vi "Inclusion_main.vi"() -> ()   [LabVIEW 2018]
uses:
  <userlib>/_OpenG.lib/numeric/numeric.llb/Random Number Within Range - DBL__ogtk.vi
  <vilib>/Analysis/NI_AALBase.lvlib
panel:
  out "Histogram Graph":T1(graph)
  out "Avg. us per sample":dbl
  in  "N samples":i32=1000
  in  "Test":bool
  in  "Type":bool
  out "Reset c3":bool
  out "Reset c2":bool
  out "Reset c1":bool
  out "Out 3":dbl
  out "Out 2":dbl
  in  "Send 3":dbl
  in  "Send 2":dbl
  out "Out 1":dbl
  in  "Send 1":dbl
  in  "Stop Button":bool
  in  "Reset all":bool
  in  "Send":bool
  in  "Reset 3":bool
  in  "Reset 2":bool
  in  "Reset 1":bool
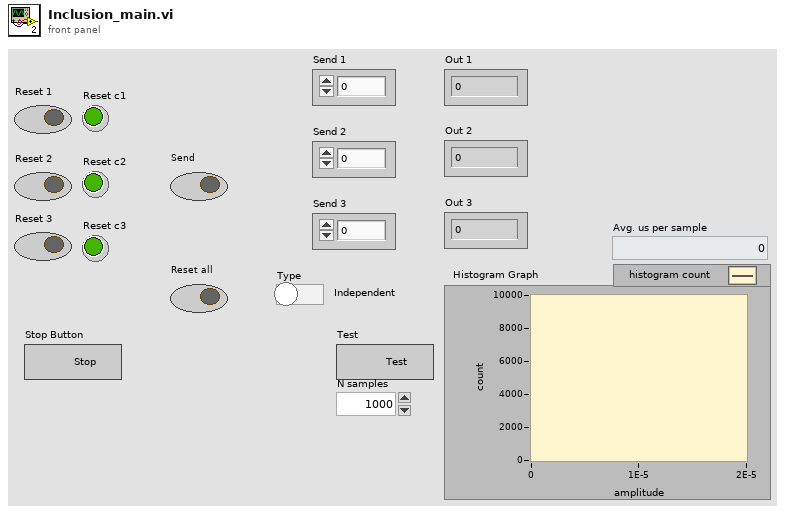
[diagram p1: front panel]
types:
  T1 = cluster{"X Values":dbl[], "Histogram: h(x)":i32[]}
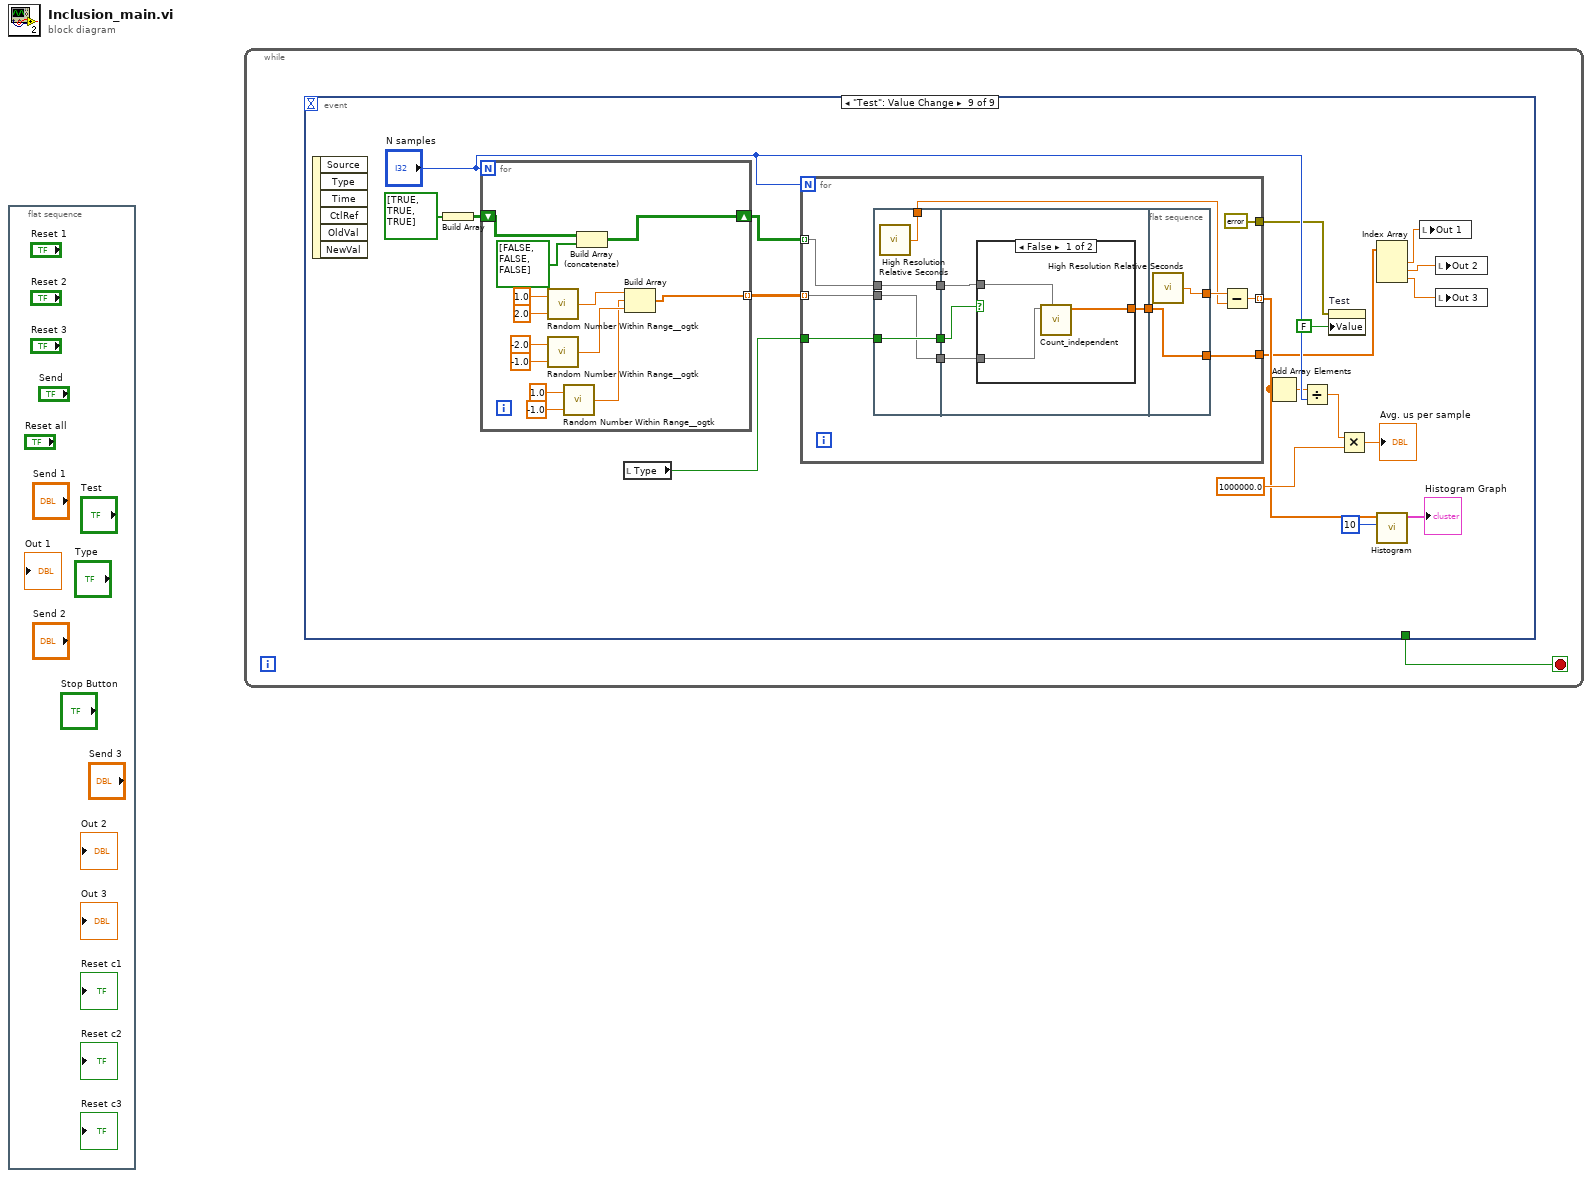
[diagram p0: block diagram]
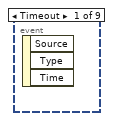
[diagram p2: hidden frame]
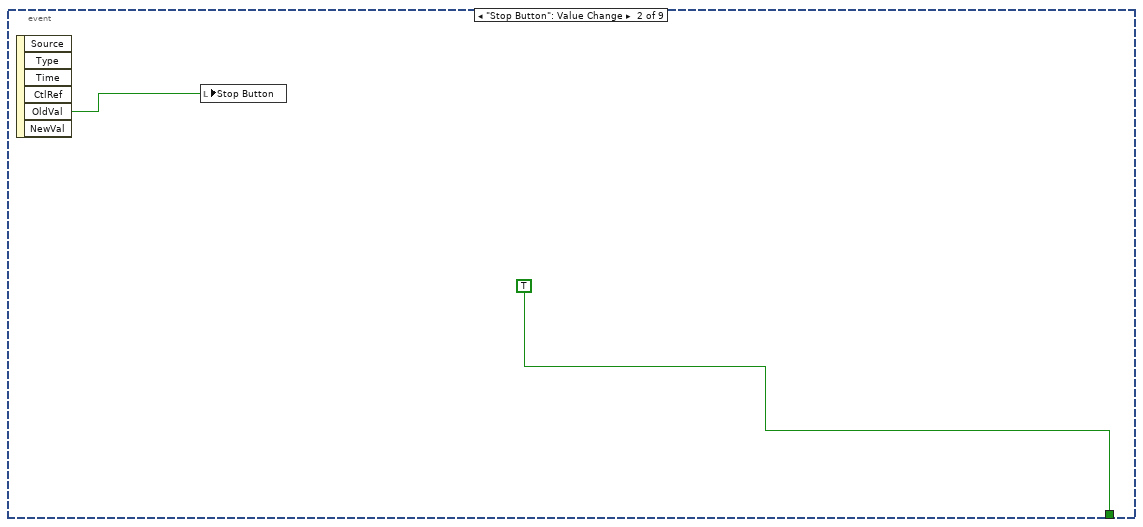
[diagram p3: hidden frame]
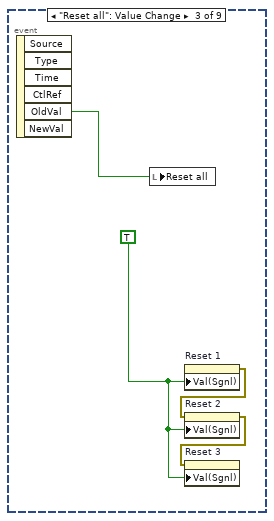
[diagram p4: hidden frame]
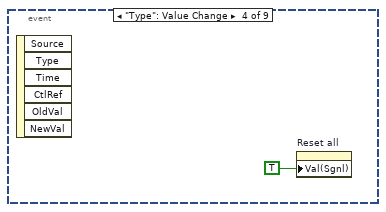
[diagram p5: hidden frame]
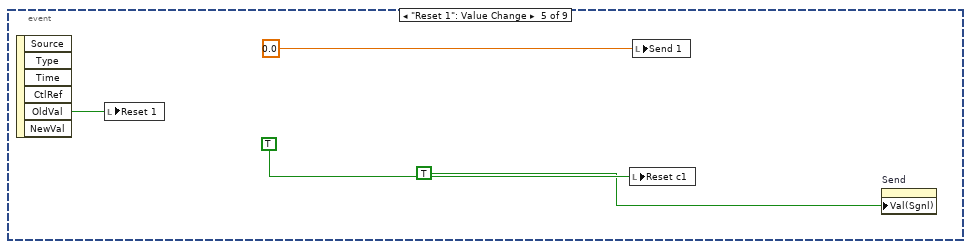
[diagram p6: hidden frame]
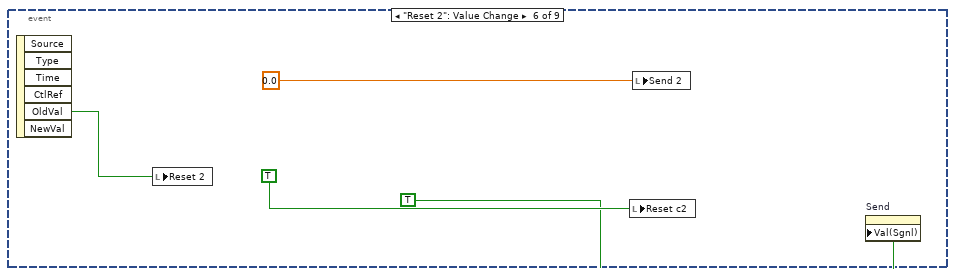
[diagram p7: hidden frame]
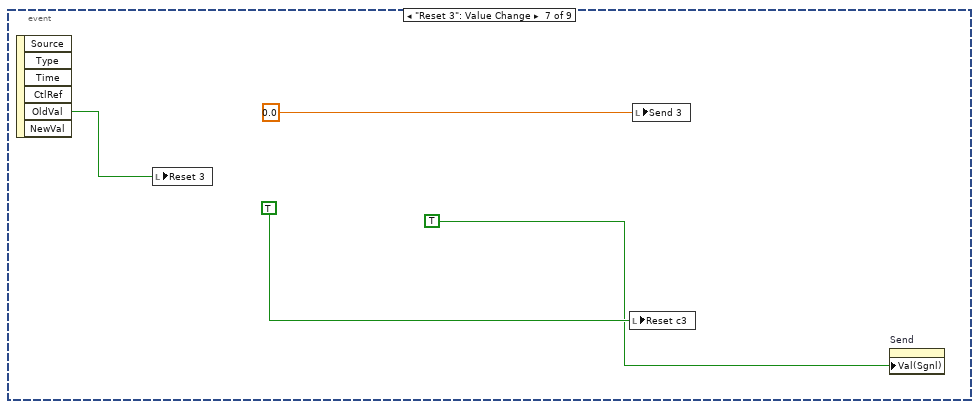
[diagram p8: hidden frame]
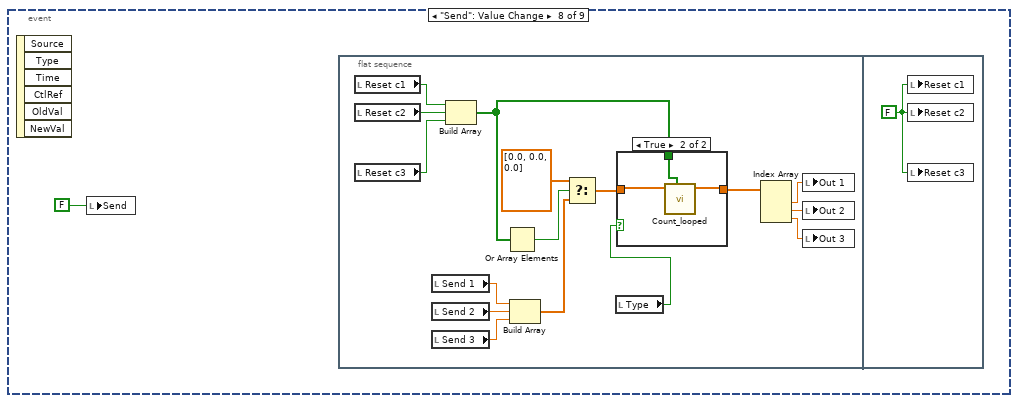
[diagram p9: hidden frame]
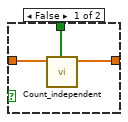
[diagram p10: hidden frame]
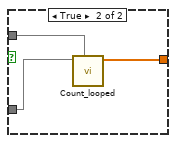
[diagram p11: hidden frame]
diagram:
  n1 = flat-sequence {
    frame #0 {
    }
  }
  n2 = while {
    stop <- w1 stop-if-true
    n3 = event shown="[8] \"Test\": Value Change" {
      selector: _ -> [_ _ _ _ _ _ _ _ _]
      dyn-events: _ -> [_ _ _ _ _ _ _ _ _]
      timeout: _ -> [_ _ _ _ _ _ _ _ _]
      tunnel: [_ TRUE _ _ _ _ _ _ _] -> w1
      event Timeout {
        n4 = event-data() -> ()  [unwired: 1 in, 3 out]
      }
      event "Stop Button": Value Change {
        n5 = event-data() -> ("OldVal"=w2:bool)  [unwired: 1 in, 5 out]
        n6 = local write "Stop Button"(w2) -> ()
      }
      event "Reset all": Value Change {
        w6 = TRUE ("Value (Signaling)")
        n7 = event-data() -> ("OldVal"=w7:bool)  [unwired: 1 in, 5 out]
        n8 = local write "Reset all"(w7) -> ()
        n9 = property on="Reset 1" class="Bool (strict)"("Val(Sgnl)"=w6) -> (error out=w5:errorcluster)  [unwired: 2 in, 1 out]
        n10 = property on="Reset 2" class="Bool (strict)"(error in=w5, "Val(Sgnl)"=w6) -> (error out=w4:errorcluster)  [unwired: 1 in, 1 out]
        n11 = property on="Reset 3" class="Bool (strict)"(error in=w4, "Val(Sgnl)"=w6) -> ()  [unwired: 1 in, 2 out]
      }
      event "Type": Value Change {
        n12 = event-data() -> ()  [unwired: 1 in, 6 out]
        n13 = property on="Reset all" class="Bool (strict)"("Val(Sgnl)"=TRUE ("Value (Signaling)")) -> ()  [unwired: 2 in, 2 out]
      }
      event "Reset 1": Value Change {
        n14 = event-data() -> ("OldVal"=w11:bool)  [unwired: 1 in, 5 out]
        n15 = local write "Reset 1"(w11) -> ()
        n16 = local write "Reset c1"(TRUE ("Reset c1")) -> ()
        n17 = local write "Send 1"(0.0 ("Send 1")) -> ()
        n18 = property on="Send" class="Bool (strict)"("Val(Sgnl)"=TRUE ("Value (Signaling)")) -> ()  [unwired: 2 in, 2 out]
      }
      event "Reset 2": Value Change {
        n19 = event-data() -> ("OldVal"=w15:bool)  [unwired: 1 in, 5 out]
        n20 = local write "Reset 2"(w15) -> ()
        n21 = local write "Reset c2"(TRUE ("Reset c2")) -> ()
        n22 = local write "Send 2"(0.0 ("Send 2")) -> ()
        n23 = property on="Send" class="Bool (strict)"("Val(Sgnl)"=TRUE ("Value (Signaling)")) -> ()  [unwired: 2 in, 2 out]
      }
      event "Reset 3": Value Change {
        n24 = event-data() -> ("OldVal"=w19:bool)  [unwired: 1 in, 5 out]
        n25 = local write "Reset 3"(w19) -> ()
        n26 = local write "Reset c3"(TRUE ("Reset c3")) -> ()
        n27 = local write "Send 3"(0.0 ("Send 3")) -> ()
        n28 = property on="Send" class="Bool (strict)"("Val(Sgnl)"=TRUE ("Value (Signaling)")) -> ()  [unwired: 2 in, 2 out]
      }
      event "Send": Value Change {
        n29 = event-data() -> ()  [unwired: 1 in, 6 out]
        n30 = local write "Send"(FALSE ("Send")) -> ()
        n31 = flat-sequence {
          frame #0 {
            n32 = local read "Reset c1"() -> (w30:bool)
            n33 = local read "Reset c2"() -> (w29:bool)
            n34 = local read "Reset c3"() -> (w28:bool)
            n35 = local read "Send 1"() -> (w37:dbl)
            n36 = local read "Send 2"() -> (w36:dbl)
            n37 = local read "Send 3"() -> (w35:dbl)
            n38 = Build Array(w30, w29, w28) -> (w27:bool[])
            n39 = Or Array Elements(Boolean array=w27) -> (logical OR=w24:bool)
            n40 = Build Array(w37, w36, w35) -> (w25:dbl[])
            n41 = Select(t=dbl[] [0.0, 0.0, 0.0], s=w24, f=w25) -> (s? t:f=w26:dbl[])
            n42 = local read "Type"() -> (w22:bool)
            n43 = case shown="True" w22 {
              tunnel: [w40 w42] -> w34
              tunnel: w27 -> [w39 w41]
              tunnel: w26 -> [w38 w43]
              frame False {
                n44 = call "Count_independent.vi"("Reset?"=w39, "Input array"=w38) -> ("Output array"=w40:dbl[])  [unwired: 9 in]
              }
              frame True {
                n45 = call "Count_looped.vi"("Reset?"=w41, "Input array"=w43) -> ("Output array"=w42:dbl[])  [unwired: 9 in]
              }
            }
            n46 = Index Array(array=w34) -> (element #1=w33:dbl, element #2=w32:dbl, element #3=w31:dbl)  [unwired: 3 in]
            n47 = local write "Out 1"(w33) -> ()
            n48 = local write "Out 2"(w32) -> ()
            n49 = local write "Out 3"(w31) -> ()
          }
          frame #1 {
            w44 = FALSE ("Reset c1")
            n50 = local write "Reset c1"(w44) -> ()
            n51 = local write "Reset c2"(w44) -> ()
            n52 = local write "Reset c3"(w44) -> ()
          }
        }
      }
      event "Test": Value Change {
        n53 = event-data() -> ()  [unwired: 1 in, 6 out]
        n54 = Build Array(bool[] [TRUE, TRUE, TRUE]) -> (w46:bool[][])
        n55 = for {
          N: "N samples" -> [_]
          tunnel: [w93] -> w51 mode=indexing
          shift-right: [w92] -> w45
          shift-left: w46 -> [w104]
          n56 = call-poly <userlib>:"Random Number Within Range__ogtk.vi"("High"=1.0, "Low"=2.0) -> ("Random Number"=w100:dbl)  [unwired: 3 in]
          n57 = call-poly <userlib>:"Random Number Within Range__ogtk.vi"("High"=-2.0, "Low"=-1.0) -> ("Random Number"=w97:dbl)  [unwired: 3 in]
          n58 = call-poly <userlib>:"Random Number Within Range__ogtk.vi"("High"=1.0, "Low"=-1.0) -> ("Random Number"=w94:dbl)  [unwired: 3 in]
          n59 = Build Array (concatenate)(w104, bool[] [FALSE, FALSE, FALSE]) -> (w92:bool[][])
          n60 = Build Array(w100, w94, w97) -> (w93:dbl[])
        }
        n61 = local read "Type"() -> (w54:bool)
        n62 = for {
          N: "N samples" -> [_]
          tunnel: [w73] -> w57 mode=indexing
          tunnel: w54 -> [w71]
          tunnel: [errorcluster {"status"=FALSE, "code"=0, "source"=""} ("error in (no error)")] -> w52
          tunnel: w51 -> [w66] mode=indexing
          tunnel: w45 -> [w68] mode=indexing
          tunnel: [w65] -> w50
          n63 = flat-sequence {
            tunnel: [w79] -> w74
            tunnel: [w78] -> w72
            tunnel: w71 -> [w78]
            tunnel: [w77] -> w69
            tunnel: w68 -> [w77]
            tunnel: [w76] -> w67
            tunnel: w66 -> [w76]
            tunnel: w72 -> [w83]
            tunnel: w69 -> [w82]
            tunnel: w67 -> [w81]
            tunnel: [w80] -> w64
            tunnel: [w91] -> w75
            tunnel: [w90] -> w65
            tunnel: w64 -> [w90]
            frame #0 {
              n64 = call <vilib>:"High Resolution Relative Seconds.vi"() -> ("relative seconds"=w79:dbl)
            }
            frame #1 {
              n65 = case shown="False" w83 {
                tunnel: w82 -> [w86 w88]
                tunnel: w81 -> [w85 w89]
                tunnel: [w84 w87] -> w80
                frame False {
                  n66 = call "Count_independent.vi"("Reset?"=w86, "Input array"=w85) -> ("Output array"=w84:dbl[])  [unwired: 9 in]
                }
                frame True {
                  n67 = call "Count_looped.vi"("Reset?"=w88, "Input array"=w89) -> ("Output array"=w87:dbl[])  [unwired: 9 in]
                }
              }
            }
            frame #2 {
              n68 = call <vilib>:"High Resolution Relative Seconds.vi"() -> ("relative seconds"=w91:dbl)
            }
          }
          n69 = Subtract(x=w75, y=w74) -> (x-y=w73:dbl)
        }
        n70 = Add Array Elements(numeric array=w57) -> (sum=w60:dbl)
        n71 = Divide(x=w60, y="N samples") -> (x/y=w61:dbl)
        n72 = property on="Test" class="Bool (strict)"(error in=w52, "Value"=FALSE ("Test")) -> ()  [unwired: 1 in, 2 out]
        n73 = Multiply(x=w61, y=1000000.0) -> (x*y=→"Avg. us per sample":dbl)
        n74 = Index Array(array=w50) -> (element #1=w49:dbl, element #2=w48:dbl, element #3=w47:dbl)  [unwired: 3 in]
        n75 = call <vilib>:"Histogram.vi"("intervals"=10, "X"=w57) -> ("Histogram Graph"=→"Histogram Graph":T1)  [unwired: 6 in, 3 out]
        n76 = local write "Out 1"(w49) -> ()
        n77 = local write "Out 2"(w48) -> ()
        n78 = local write "Out 3"(w47) -> ()
      }
    }
  }
